vi "Create.vi"(8 "Error In":errorcluster, 10 "ICommunicate":refnum<class "ICommunicate.lvclass">) -> (0 "Error Out":errorcluster, 3 "SDO Manager":refnum<class "SDO Manager.lvclass">)   [LabVIEW 2020, in "SDO Manager.lvlib" / "SDO Manager.lvclass"]
uses:
  SDO Manager.lvclass
  SDO Manager.lvclass/SDO Manager.ctl
  SDO Manager Worker/SDO Manager Worker.lvclass
  C:/Program Files/National Instruments/LabVIEW 2026/vi.lib/ActorFramework/Actor/Actor.lvclass
  D:/git/CANopen-LabVIEW/source/SDO Manager/SDO Manager Worker/SDO Manager Worker.lvclass
  SDO Transfer/SDO Transfer.lvclass
  <vilib>/ActorFramework/Actor/Actor.lvclass
  HAL/Source/Interfaces/ICommunicate/ICommunicate.lvclass
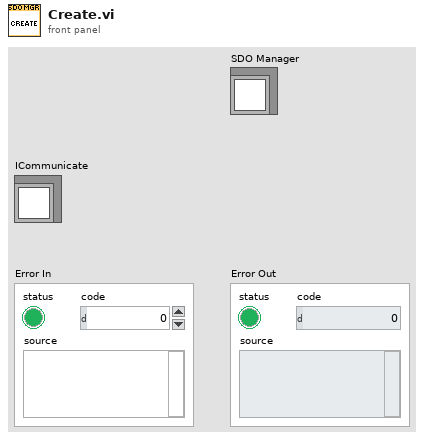
[diagram p1: front panel]
types:
  T1 = map{string, refnum<class "SDO Transfer.lvclass">}
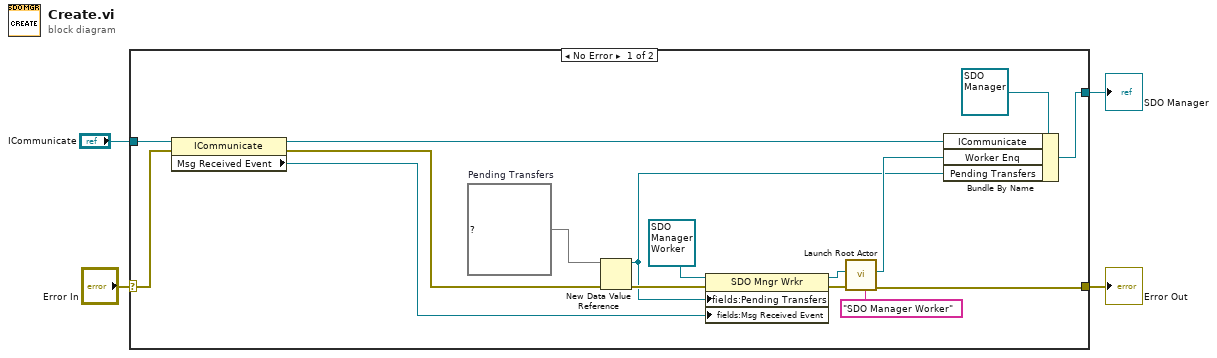
[diagram p0: block diagram]
diagram:
  n1 = case shown="No Error" "Error In" {
    selector: "Error In" -> [w14 w21]
    tunnel: [w16 w21] -> w3
    tunnel: [w13 _] -> w2
    tunnel: "ICommunicate" -> [w7 _]
    frame No Error {
      w20 = T1 {}  # Pending Transfers
      n2 = property class="ICommunicate"(reference=w7, error in=w14) -> (reference out=w6:refnum<class "ICommunicate.lvclass">, error out=w8:errorcluster, "Msg Received Event"=w5:refnum<user-event>)
      n3 = New Data Value Reference(data value=w20, error in=w8) -> (data value reference=w9:refnum<data-value>, error out=w17:errorcluster)
      n4 = property class="SDO Mngr Wrkr"(reference=refnum<class "SDO Manager Worker.lvclass"> refnum ("CANopen Master:SDO Mngr Wrkr"), error in=w17, "fields:Pending Transfers"=w9, "fields:Msg Received Event"=w5) -> (reference out=w10:refnum<class "SDO Manager Worker.lvclass">, error out=w12:errorcluster)
      n5 = call <vilib>:"Launch Root Actor.vi"("Debug Alias"="SDO Manager Worker", "error in (no error)"=w12, "Actor"=w10) -> ("error out"=w16:errorcluster, "Actor's Enqueuer"=w18:refnum<class "Message Enqueuer.lvclass">)  [unwired: 7 in]
      n6 = Bundle By Name(cluster=refnum<class "SDO Manager.lvclass"> refnum ("reference out"), "ICommunicate"=w6, "Worker Enq"=w18, "Pending Transfers"=w9) -> (w13:refnum<class "SDO Manager.lvclass">)
    }
    frame Error {
      # "VI-TechBaseTemplate_Simple_4x4x4"
    }
  }
  "Error Out" <- w3
  "SDO Manager" <- w2
